vi "External_Move.vi"(8 "error in (no error)":errorcluster, 11 "TranslationStageUI in":refnum<class "TranslationStageUI.lvclass">) -> (0 "error out":errorcluster, 3 "TranslationStageUI out":refnum<class "TranslationStageUI.lvclass">)   [LabVIEW 2023, in "TranslationStageUI.lvclass"]
uses:
  TranslationStageUI.lvclass
  TranslationStageUI.lvclass/TranslationStageUI.ctl
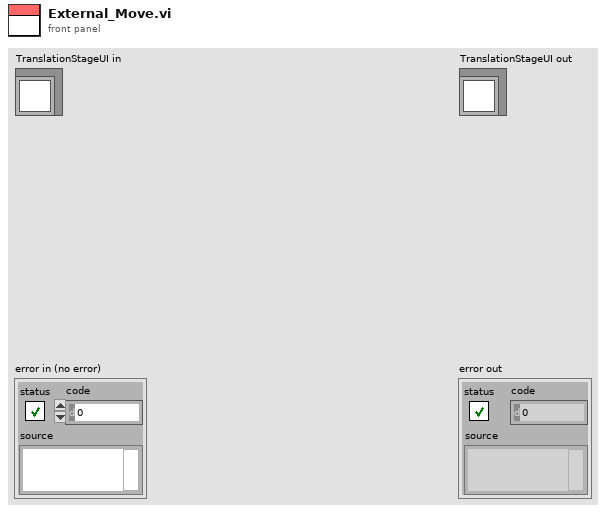
[diagram p1: front panel]
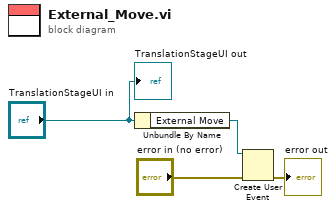
[diagram p0: block diagram]
diagram:
  n1 = Unbundle By Name("TranslationStageUI in") -> ("External Move"=w1:refnum<user-event>)
  n2 = Create User Event(user event datatype=w1, error in="error in (no error)") -> (error out=→"error out":errorcluster)  [unwired: 1 out]
  "TranslationStageUI out" <- "TranslationStageUI in"
